vi "Fetch Power Sensor.vi"(8 "error in (no error)":errorcluster, 10 "Instance (1)":i32=1 format="%.0g", 11 "VISA resource name":refnum<visa-resource-name>) -> (0 "error out":errorcluster, 1 "Power":dbl[](array[numeric]) format="%^.3e", 2 "Reliability":i32, 3 "VISA resource name out":refnum<visa-resource-name>, 4 "Elapsed Statistics":i32)   [LabVIEW 2015, in "Rohde&Schwarz CMXP GPRF.lvlib"]
doc: "Returns the results of the current measurement cycle (single shot measurement) after they are valid. FETCh... must be used after the measurement has been started (INITiate..., measurement states RUN or RDY).\n\nAttribute:\nRSCMXPGPRF_ATTR_FETCH_POWER_SENSOR\n\nRemote-control command:\nFETCh:GPRF:MEAS<i>:EPSensor?"
uses:
  <instrlib>/Rohde&Schwarz CMXP GPRF/Rohde&Schwarz CMXP GPRF.lvlib
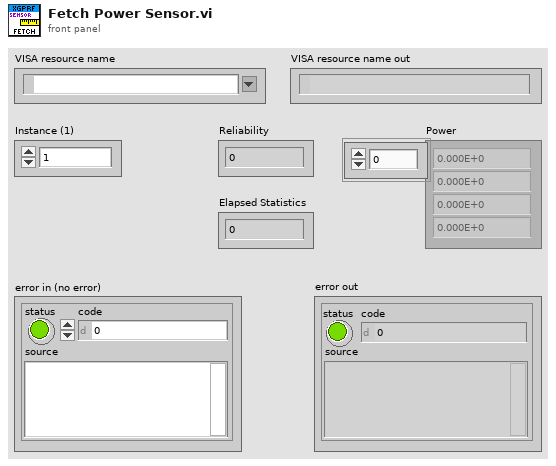
[diagram p1: front panel]
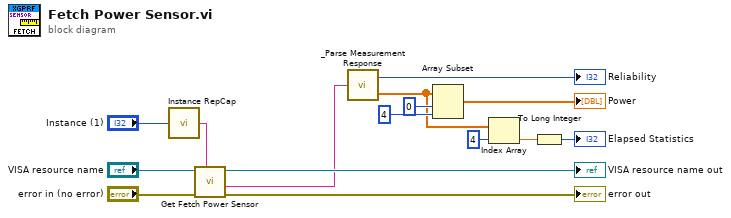
[diagram p0: block diagram]
diagram:
  n1 = call <instrlib>:"Instance RepCap.vi"("instance  in"="Instance (1)") -> ("instance out"=w15:string)
  n2 = call "Get Fetch Power Sensor"("Repeated Capabilities"=w15, "error in (no error)"="error in (no error)", "instrument handle"="VISA resource name") -> ("error out"=→"error out":errorcluster, "Fetch Power Sensor"=w1:string, "instrument handle out"=→"VISA resource name out":refnum<visa-resource-name>)  [unwired: 6 in]
  n3 = call <instrlib>:"_Parse Measurement Response.vi"("String In"=w1) -> ("Reliability"=→"Reliability":i32, "Data"=w5:dbl[])
  n4 = Array Subset(array=w5, index=0, length=4) -> (→"Power":dbl[])
  n5 = Index Array(array=w5, index=4) -> (element=w6:dbl)
  n6 = To Long Integer(number=w6) -> (32bit integer=→"Elapsed Statistics":i32)
